vi "GetOnboardAcceleration.vi"(11 "packet in":u8[](array[numeric])) -> (1 "accZ":i16, 2 "accY":i16, 3 "accX":i16)   [LabVIEW 2018]
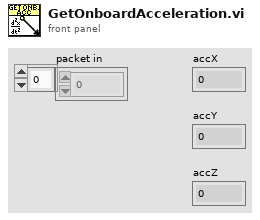
[diagram p1: front panel]
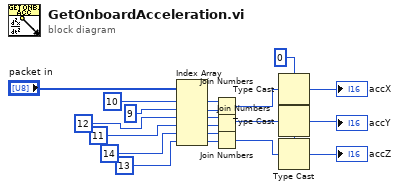
[diagram p0: block diagram]
diagram:
  w14 = i16 0 ("index")
  n1 = Index Array(array="packet in", index #1=10 ("index"), index #2=9 ("index"), index #3=12 ("index"), index #4=11 ("index"), index #5=14 ("index"), index #6=13 ("index")) -> (element #1=w8:u8, element #2=w9:u8, element #3=w10:u8, element #4=w11:u8, element #5=w12:u8, element #6=w13:u8)
  n2 = Join Numbers(hi=w8, lo=w9) -> ((hi.lo)=w18:u16)
  n3 = Join Numbers(hi=w11, lo=w10) -> ((hi.lo)=w19:u16)
  n4 = Join Numbers(hi=w13, lo=w12) -> ((hi.lo)=w20:u16)
  n5 = Type Cast(type=w14, x=w18) -> (*(type *) &x=→"accX":i16)
  n6 = Type Cast(type=w14, x=w19) -> (*(type *) &x=→"accY":i16)
  n7 = Type Cast(type=w14, x=w20) -> (*(type *) &x=→"accZ":i16)
